vi "Trigger.vi"() -> ()   [LabVIEW 2021]
panel:
  in  "repeat count":i32(knob)=3 scale=0.0..5.0
  out "trial":i32
  out "COUNTDOWN":i32
  in  "stop":bool
  in  "OK Button":bool
  out "Boolean":bool
  # "Trial Number :"
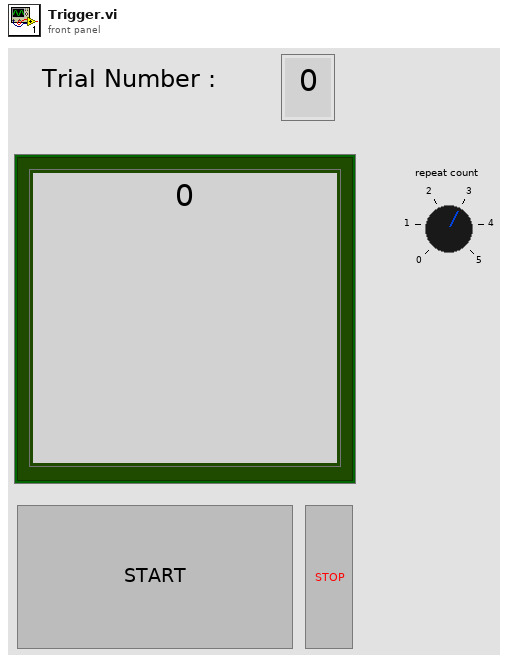
[diagram p1: front panel]
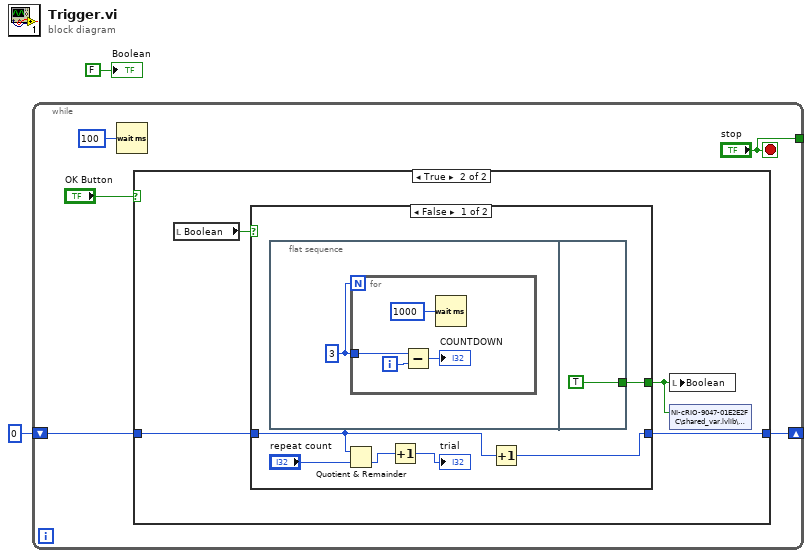
[diagram p0: block diagram]
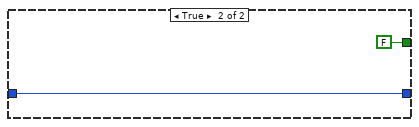
[diagram p3: hidden frame]
diagram:
  n1 = while {
    tunnel: ["stop"] -> _
    shift-right: [w3] -> _
    shift-left: 0 ("y") -> [w4]
    stop <- "stop" stop-if-true
    n2 = Wait (ms)(milliseconds to wait=u32 100) -> ()  [unwired: 1 out]
    n3 = case shown="True" "OK Button" {
      tunnel: w4 -> [w8 w10]
      tunnel: [w8 w9] -> w3
      frame False {
      }
      frame True {
        n4 = local read "Boolean"() -> (w11:bool)
        n5 = case shown="False" w11 {
          tunnel: [w18 FALSE ("Trigger")] -> w12
          tunnel: w10 -> [w16 w25]
          tunnel: [w15 w25] -> w9
          frame False {
            n6 = flat-sequence {
              tunnel: [TRUE ("Trigger")] -> w18
              frame #0 {
                w19 = 3 ("y")
                n7 = for {
                  N: w19 -> [_]
                  tunnel: w19 -> [w21]
                  i -> [w23]
                  n8 = Subtract(x=w21, y=w23) -> (x-y=→"COUNTDOWN":i32)
                  n9 = Wait (ms)(milliseconds to wait=u32 1000) -> ()  [unwired: 1 out]
                }
              }
              frame #1 {
              }
            }
            n10 = Quotient & Remainder(x=w16, y="repeat count") -> (floor(x/y)=w14:i32)  [unwired: 1 out]
            n11 = Increment(x=w14) -> (x+1=→"trial":i32)
            n12 = Increment(x=w16) -> (x+1=w15:i32)
          }
          frame True {
          }
        }
        n13 = local write "Boolean"(w12) -> ()
        n14 = shared-variable "NI-cRIO-9047-01E2E2FC\\shared_var.lvlib\\Trigger"(w12) -> ()  [unwired: 1 in, 1 out]
      }
    }
  }
  "Boolean" <- FALSE ("Boolean")
